vi "Uninit SignalWithAlarm.vi"(8 "error in (no error)":errorcluster, 11 "SignalWithAlarm in":refnum<class "SignalWithAlarm.lvclass">) -> (0 "error out":errorcluster, 3 "SignalWithAlarm out":refnum<class "SignalWithAlarm.lvclass">)   [LabVIEW 2016, in "SignalWithAlarm.lvclass"]
uses:
  SignalWithAlarm.lvclass
  SignalWithAlarm.lvclass/SignalWithAlarm.ctl
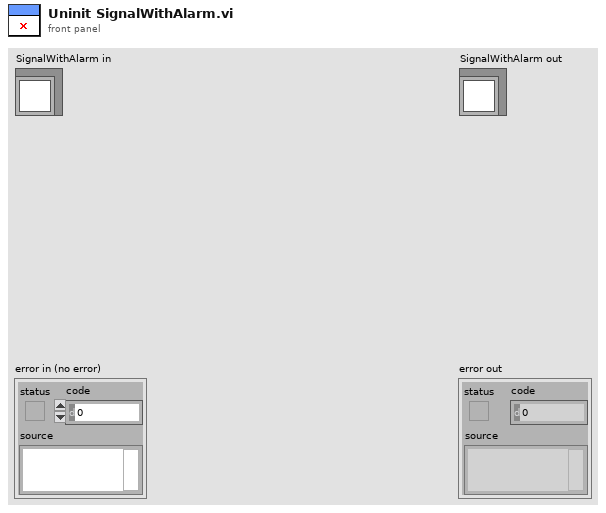
[diagram p1: front panel]
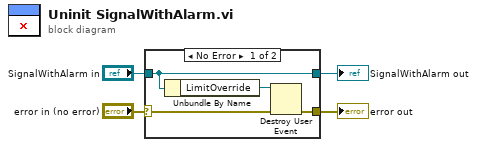
[diagram p0: block diagram]
diagram:
  n1 = case shown="No Error" "error in (no error)" {
    selector: "error in (no error)" -> [w7 w10]
    tunnel: [w6 w10] -> w3
    tunnel: [w5 w9] -> w1
    tunnel: "SignalWithAlarm in" -> [w5 w9]
    frame No Error {
      n2 = Unbundle By Name(w5) -> ("LimitOverride"=w8:refnum<user-event>)
      n3 = Destroy User Event(user event=w8, error in=w7) -> (error out=w6:errorcluster)
    }
    frame Error {
    }
  }
  "error out" <- w3
  "SignalWithAlarm out" <- w1
